vi "Enable.vi"(8 "error in (no error)":errorcluster, 10 "Enable?":bool, 11 "reference in":refnum<class "DUT_Handler_Simple.lvclass">) -> (0 "error out":errorcluster, 3 "reference in":refnum<class "DUT_Handler_Simple.lvclass">)   [LabVIEW 2022 SP3, in "DUT_Handler_Simple.lvlib" / "DUT_Handler_Simple.lvclass"]
uses:
  DUT_Handler_Simple.lvclass
  Components/DUT_Handler_Base.lvlibp/EventData.ctl
  Components/DUT_Handler_Base.lvlibp/Action.ctl
  Components/DUT_Handler_Base.lvlibp/DUT_Handler_Base.lvclass
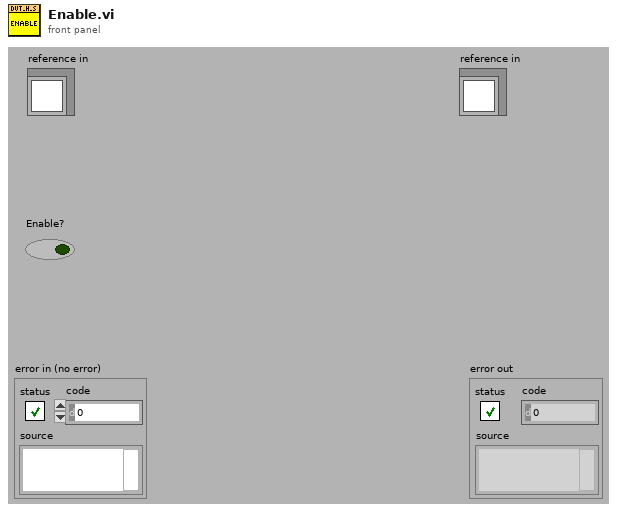
[diagram p1: front panel]
types:
  T1 = typedef "DUT_Handler_Base.lvlibp/DUT_Handler_Base.lvclass/Action.ctl" = enum16{"Load", "Cancel", "MoveIn", "MoveOut", "Abort", "Msg", "Enabled", "Disabled", "Fault", "Shutdown"}
  T2 = typedef "DUT_Handler_Base.lvlibp/DUT_Handler_Base.lvclass/EventData.ctl" = cluster{"Action":enum16{"Load", "Cancel", "MoveIn", "MoveOut", "Abort", "Msg", "Enabled", "Disabled", "Fault", "Shutdown"}, "SN":string, "BN":string, "DUT__ID":u32, "Message":string, "From":string, "To":string}
  T3 = typedef "DUT_Handler_Simple.lvlib/DUT_Handler_Simple.lvclass/ObjectAttributes.ctl" = cluster{"Config":T4, "event_data":T2, "Enabled":bool, "Barcode_Reader":refnum<class "Barcode_Reader_Base.lvclass">}
  T4 = typedef "DUT_Handler_Simple.lvlib/DUT_Handler_Simple.lvclass/Config.ctl" = cluster{"default":string}
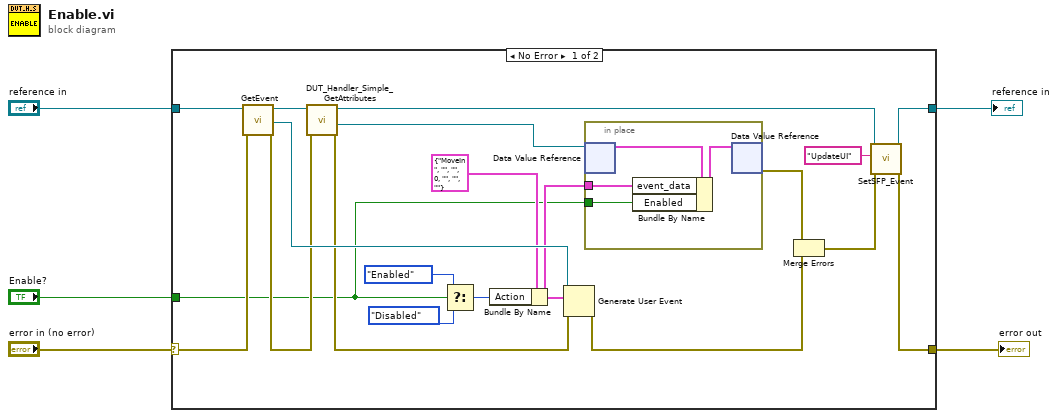
[diagram p0: block diagram]
diagram:
  n1 = case shown="No Error" "error in (no error)" {
    selector: "error in (no error)" -> [w24 w31]
    tunnel: [w12 w31] -> w4
    tunnel: [w13 w30] -> w2
    tunnel: "reference in" -> [w25 w30]
    tunnel: "Enable?" -> [w16 _]
    frame No Error {
      n2 = call-dynamic "GetEvent.vi"("error in (no error)"=w24, "reference in"=w25) -> ("error out"=w21:errorcluster, "DUT_Handler"=w23:refnum<user-event>, "reference in"=w22:refnum<class "DUT_Handler_Simple.lvclass">)  [unwired: 6 in]
      n3 = call "DUT_Handler_Simple_GetAttributes.vi"("error in (no error)"=w21, "reference in"=w22) -> ("error out"=w20:errorcluster, "DataRef"=w19:refnum<data-value>, "reference out"=w14:refnum<class "DUT_Handler_Simple.lvclass">)  [unwired: 6 in, 1 out]
      n4 = Select(t=Action."Enabled" ("Action"), s=w16, f=Action."Disabled" ("Action")) -> (s? t:f=w6:T1)
      n5 = Bundle By Name(cluster=T2 {"Action"=enum."MoveIn", "SN"="", "BN"="", "DUT__ID"=0, "Message"="", "From"="", "To"=""} ("event_data"), "Action"=w6) -> (w17:T2)
      n6 = Generate User Event(user event=w23, event data cluster=w17, error in=w20) -> (error out=w10:errorcluster)  [unwired: 1 in, 1 out]
      n7 = in-place {
        in-place-border: w17 -> [w27]
        in-place-border: w16 -> [w26]
        n8 = in-place-dvr #1(w19) -> (w29:T3)  [unwired: 1 out]
        n9 = Bundle By Name(cluster=w29, "event_data"=w27, "Enabled"=w26) -> (w28:T3)
        n10 = in-place-dvr #1(w28) -> (w11:errorcluster)  [unwired: 1 out]
      }
      n11 = Merge Errors(w11, w10) -> (w9:errorcluster)
      n12 = call-dynamic "SetSFP_Event.vi"("error in (no error)"=w9, "msg"="UpdateUI", "reference in"=w14) -> ("error out"=w12:errorcluster, "reference out"=w13:refnum<class "DUT_Handler_Simple.lvclass">)  [unwired: 7 in]
    }
    frame Error {
    }
  }
  "error out" <- w4
  "reference in" <- w2
